vi "editscenario Save Scenario.vi"(6 "User Information":T4, 8 "error in (no error)":errorcluster, 9 "Save POST":T5, 10 "scenarioId (\"\")":string, 11 "Connection Refnum":T6) -> (0 "error out":errorcluster, 2 "New Scenario":T1, 3 "Connection Refnum":T6)   [LabVIEW 2011]
uses:
  Summitek EXT/ODBC/SQL Controls/Connection Refnum.ctl
  ITK EXT/utils/keyedarr.llb/Keyed Array.ctl
  server/database/Users/User Record.ctl
  server/database/Scenarios/Scenario Record.ctl
  server/database/Scenarios/Conditions/Condition Record.ctl
  server/database/Scenarios/Conditions/Condition Operators.ctl
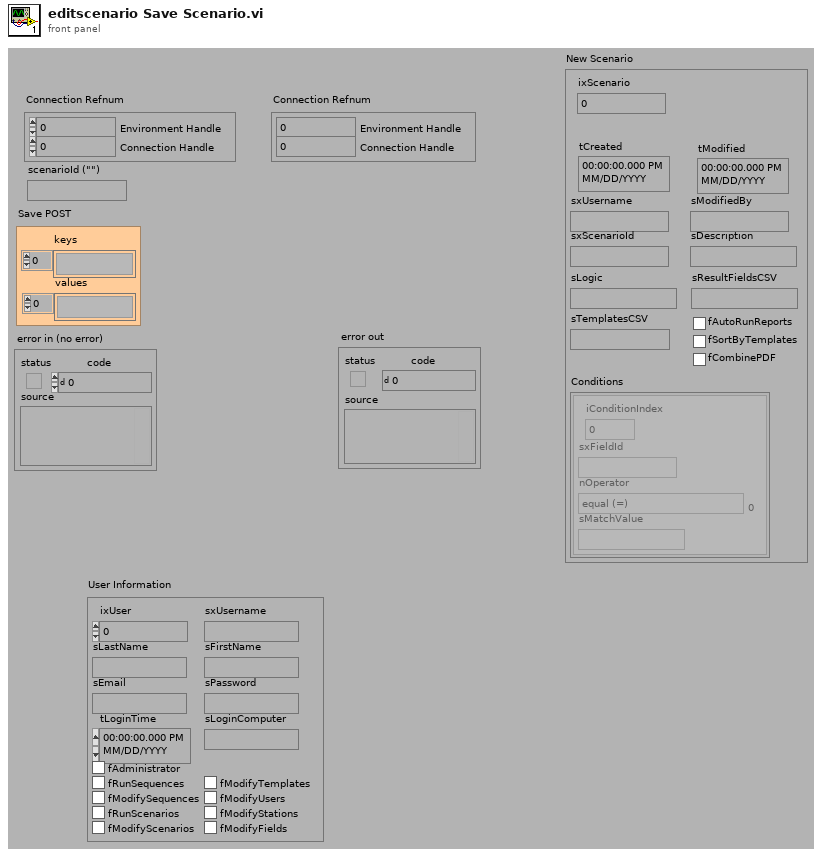
[diagram p1: front panel]
types:
  T1 = typedef "Scenario Record.ctl" = cluster{"ixScenario":i32, "tCreated":timestamp, "tModified":timestamp, "sxUsername":string, "sModifiedBy":string, "sxScenarioId":string, "sDescription":string, "sLogic":string, "sResultFieldsCSV":string, "sTemplatesCSV":string, "fAutoRunReports":bool, "fSortByTemplates":bool, "fCombinePDF":bool, "Conditions":T2[]}
  T2 = typedef "Condition Record.ctl" = cluster{"iConditionIndex":i32, "sxFieldId":string, "nOperator":T3, "sMatchValue":string}
  T3 = typedef "Condition Operators.ctl" = enum16{"equal (=)", "not equal (\\u2260)", "less than (<)", "less than or equal (\\u2264)", "greater than (>)", "greater than or equal (\\u2265)", "contains", "does not contain"}
  T4 = typedef "User Record.ctl" = cluster{"ixUser":i32, "sxUsername":string, "sLastName":string, "sFirstName":string, "sEmail":string, "sPassword":string, "tLoginTime":timestamp, "sLoginComputer":string, "fAdministrator":bool, "fRunSequences":bool, "fModifySequences":bool, "fRunScenarios":bool, "fModifyScenarios":bool, "fModifyTemplates":bool, "fModifyUsers":bool, "fModifyStations":bool, "fModifyFields":bool}
  T5 = typedef "Keyed Array.ctl" = cluster{"keys":string[], "values":string[]}
  T6 = typedef "Connection Refnum.ctl" = cluster{"Environment Handle":i32, "Connection Handle":i32}
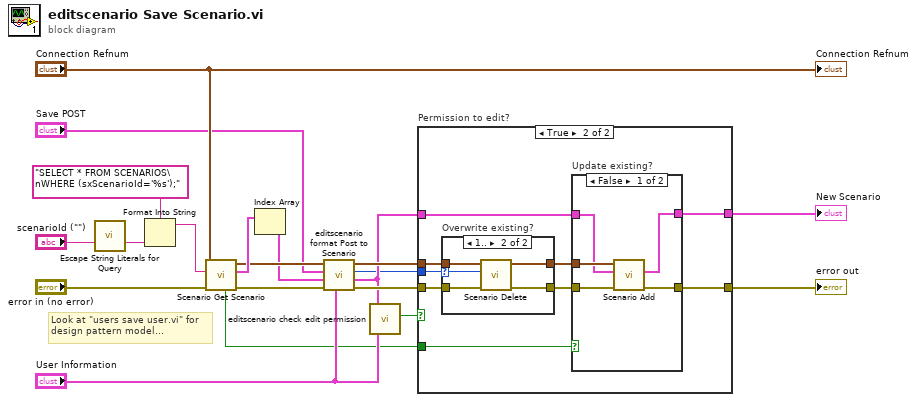
[diagram p0: block diagram]
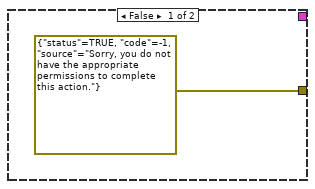
[diagram p2: hidden frame]
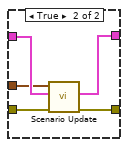
[diagram p4: hidden frame]
diagram:
  # "Look at \"users save user.vi\" for\ndesign pattern model..."
  n1 = call "Escape String Literals for Query.vi"("String"="scenarioId (\"\")") -> ("escaped String"=w11:string)  [unwired: 1 in, 13 out]
  n2 = Format Into String(format string="SELECT * FROM SCENARIOS\nWHERE (sxScenarioId='%s');", w11) -> (resulting string=w18:string)  [unwired: 2 in, 1 out]
  n3 = call "Scenario Get Scenario.vi"("error in (no error)"="error in (no error)", "Query"=w18, "Connection Refnum"="Connection Refnum") -> ("error out"=w14:errorcluster, "Scenarios"=w16:T1[], "Connection Refnum"=w8:T6, "Data Present?"=w1:bool)  [unwired: 5 out]
  n4 = Index Array(array=w16) -> (element=w7:T1)  [unwired: 1 in]
  n5 = call "editscenario format Post to Scenario.vi"("User Information"="User Information", "error in (no error)"=w14, "Scenario (none)"=w7, "Save POST"="Save POST", "Connection Ref"=w8) -> ("error out"=w13:errorcluster, "new Scenario"=w4:T1, "Overwrite ixScenario"=w3:i32, "dup Connection Ref"=w5:T6)  [unwired: 3 out]
  n6 = call "editscenario check edit permission.vi"("User Information"="User Information", "Scenario Record"=w4) -> ("Okay to Edit?"=w2:bool)  [unwired: 5 out]
  n7 = case "Permission to edit?" shown="True" w2 {
    tunnel: w13 -> [_ w24]
    tunnel: [errorcluster {"status"=TRUE, "code"=-1, "source"="Sorry, you do not have the appropriate permissions to complete this action."} ("error out") w30] -> w15
    tunnel: w5 -> [_ w25]
    tunnel: w4 -> [_ w28]
    tunnel: [_ w29] -> w9
    tunnel: w3 -> [_ w26]
    tunnel: w1 -> [_ w27]
    frame False {
    }
    frame True {
      n8 = case "Overwrite existing?" shown="1.." w26 {
        selector: w26 -> [_ w33]
        tunnel: [w32 w37] -> w23
        tunnel: [w31 w36] -> w22
        tunnel: w24 -> [w31 w34]
        tunnel: w25 -> [w32 w35]
        frame 0, Default {
        }
        frame 1.. {
          n9 = call "Scenario Delete.vi"("error in (no error)"=w34, "ixScenario (0)"=w33, "Connection Refnum"=w35) -> ("error out"=w36:errorcluster, "Connection Refnum"=w37:T6)  [unwired: 7 out]
        }
      }
      n10 = case "Update existing?" shown="False" w27 {
        tunnel: [w40 w47] -> w30
        tunnel: [w38 w46] -> w29
        tunnel: w28 -> [w39 w45]
        tunnel: w23 -> [w42 w44]
        tunnel: w22 -> [w41 w43]
        frame False {
          n11 = call "Scenario Add.vi"("error in (no error)"=w41, "Scenario Record"=w39, "Connection Refnum"=w42) -> ("error out"=w40:errorcluster, "New Scenario"=w38:T1)  [unwired: 7 out]
        }
        frame True {
          n12 = call "Scenario Update.vi"("error in (no error)"=w43, "Scenario (none)"=w45, "Connection Refnum"=w44) -> ("error out"=w47:errorcluster, "dup Scenario"=w46:T1)  [unwired: 7 out]
        }
      }
    }
  }
  "error out" <- w15
  "New Scenario" <- w9
  "Connection Refnum" <- "Connection Refnum"
